vi "Within Limits.vi"(8 "error in (no error)":errorcluster, 10 "Limits in":cluster{"Min":i64, "Max":i64}, 11 "X":refnum<class "High Res Arithmetic.lvclass">) -> (0 "error out":errorcluster, 2 "Within Limits?":bool)   [LabVIEW 2021, in "High Res Arithmetic.lvclass"]
uses:
  Trace.lvclass/Trace.ctl
  High Res Arithmetic/High Res Arithmetic.lvclass
  High Res Arithmetic/High Res Arithmetic.lvclass/High Res Arithmetic.ctl
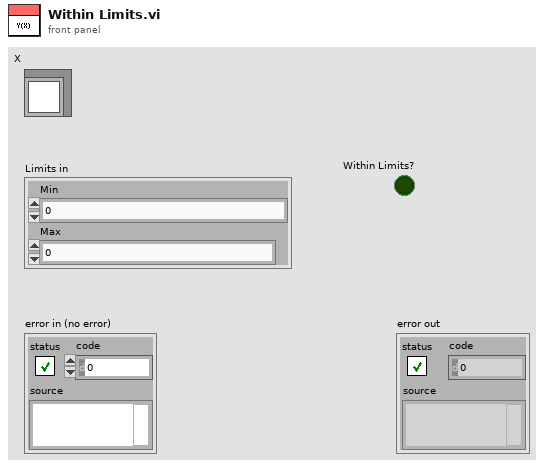
[diagram p1: front panel]
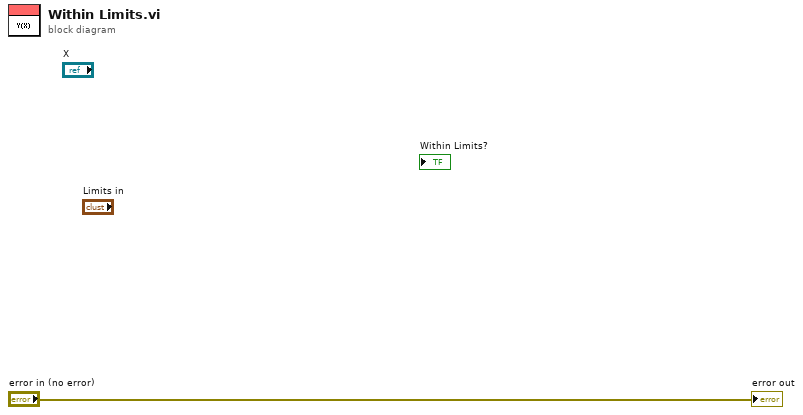
[diagram p0: block diagram]
diagram:
  "error out" <- "error in (no error)"
